vi "Update TDMS File.vi"(6 "Data Point":dbl, 8 "error in":errorcluster, 11 "Path":path) -> (0 "error out":errorcluster)   [LabVIEW 2009]
doc: "This sub VI is called by the TDMS report class.\n\nAAL 9/09"
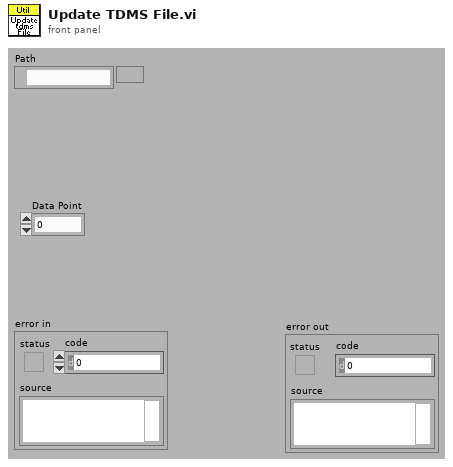
[diagram p1: front panel]
types:
  T1 = enum16{"open", "open or create", "create or replace", "create", "open (read-only)"}
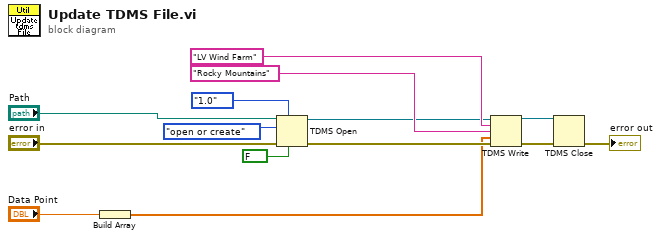
[diagram p0: block diagram]
diagram:
  n1 = Build Array("Data Point") -> (w1:dbl[])
  n2 = TDMS Open(6:FALSE ("disable buffering (T)"), 7:enum16{"1.0", "2.0"}."1.0" ("file format version (2.0)"), 8:"error in", 10:T1."open or create" ("operation (0:open)"), 11:"Path") -> (0:w3:errorcluster, 3:w4:refnum<k34>)  [unwired: 1 in]
  n3 = TDMS Write(0:w4, 5:"LV Wind Farm", 7:"Rocky Mountains", 9:w1, 11:w3) -> (4:w12:refnum<k34>, 15:w11:errorcluster)  [unwired: 1 in, 2 out]
  n4 = TDMS Close(8:w11, 11:w12) -> (0:→"error out":errorcluster)
